vi "Linearisation.vi"(9 "Array distance, D (um)":dbl, 10 "x point 2":dbl, 11 "x point 1":dbl) -> (3 "Corrected angle":dbl format="%.9g")   [LabVIEW 2022 SP3]
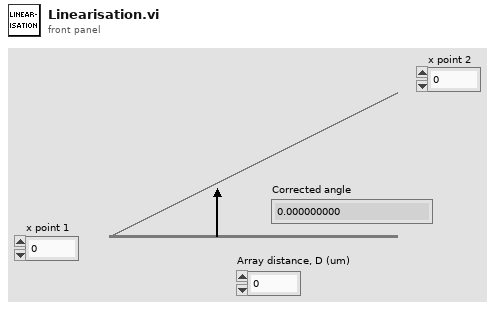
[diagram p1: front panel]
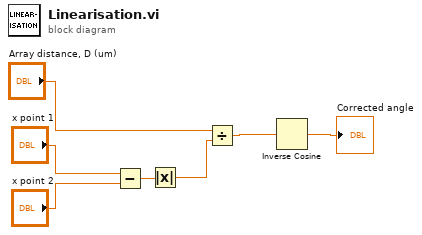
[diagram p0: block diagram]
diagram:
  n1 = Subtract(x="x point 1", y="x point 2") -> (x-y=w3:dbl)
  n2 = Absolute Value(x=w3) -> (abs(x)=w1:dbl)
  n3 = Divide(x="Array distance, D (um)", y=w1) -> (x/y=w7:dbl)
  n4 = Inverse Cosine(1:w7) -> (0:→"Corrected angle":dbl)
